vi "Abort.vi"(8 "error in (no error)":errorcluster, 11 "AcPwrSim in":refnum<class "AcPwrSimBase.lvclass">) -> (0 "error out":errorcluster, 3 "AcPwrSim out":refnum<class "AcPwrSimBase.lvclass">)   [LabVIEW 2018, in "AcPwrPlugins.lvlib" / "AcPwrSimBase.lvclass"]
uses:
  AcPwrSimBase.lvclass
  Database/DatabaseBaseClass/DatabaseBaseClass.lvclass
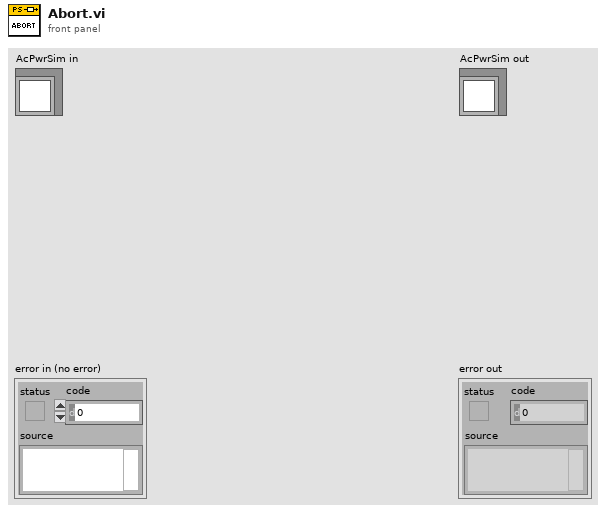
[diagram p1: front panel]
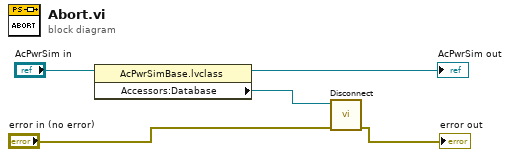
[diagram p0: block diagram]
diagram:
  n1 = property class="AcPwrSimBase.lvclass"(reference="AcPwrSim in") -> ("Accessors:Database"=w1:refnum<class "DatabaseBaseClass.lvclass">)  [unwired: 1 in, 2 out]
  n2 = call-dynamic "Disconnect.vi"("error in (no error)"="error in (no error)", "DatabaseBaseClass in"=w1) -> ("error out"=→"error out":errorcluster)  [unwired: 8 in, 1 out]
  "AcPwrSim out" <- "AcPwrSim in"
